vi "MB Serial Example Slave MK2.vi"() -> ()   [LabVIEW 2021]
uses:
  API/Wrapper/API Main.lvlib
  API/Slave/Modbus Slave.lvclass
  API/Wrapper/Create Serial Slave.vi
  Data Model/Identification Parameters.ctl
  Data Model/Device Data Model.lvclass
  Master Function Definition/Read Device ID code.ctl
panel:
  in  "VISA resource name":refnum<visa-resource-name>="COM8"
  in  "HR to write":u16[](array[numeric])=[1, 65535, 40000, 20000]
  in  "Set HR":bool
  in  "Set IR":bool
  in  "IR to write":u16[](array[numeric])=[1, 65535, 40000, 20000]
  in  "IR 6":u16
  in  "Set !":bool
  in  "! status":u8=1
  in  "Set Coils":bool
  in  "Set DI":bool
  in  "DI to write":bool[](array[boolean])=[FALSE, TRUE, FALSE, TRUE]
  in  "coils to write":bool[](array[boolean])=[FALSE, TRUE, FALSE, TRUE]
  in  "set objects":bool
  in  "Objects In":T1[](array[typedef])=[{"Object ID"=0, "Value"="National instruments"}, {"Object ID"=1, "Value"="42"}, {"Object ID"=2, "Value"="1.0.0"}] {"Object ID" format="%x"}
  in  "Coil 6":bool
  out "exception status":u8=1
  out "register values":u16[](array[numeric])=[1, 1, 65535, 40000, 20000, 6]
  out "discrete inputs":bool[](array[boolean])=[FALSE, FALSE, TRUE, FALSE, TRUE, TRUE]
  in  "Read Device ID code":T2
  out "Objects":T1[](array[typedef])=[{"Object ID"=0, "Value"="National instruments"}, {"Object ID"=1, "Value"="42"}, {"Object ID"=2, "Value"="1.0.0"}] {"Object ID" format="%x"}
  in  "Object Id":u8 format="%02x"
  out "holding reg":u16[](array[numeric])=[1, 1, 65535, 40000, 20000, 6]
  out "error out":errorcluster
  in  "stop":bool
  out "Coils":bool[](array[boolean])=[FALSE, FALSE, TRUE, FALSE, TRUE, TRUE] caption="Coils (Master can write coils)"
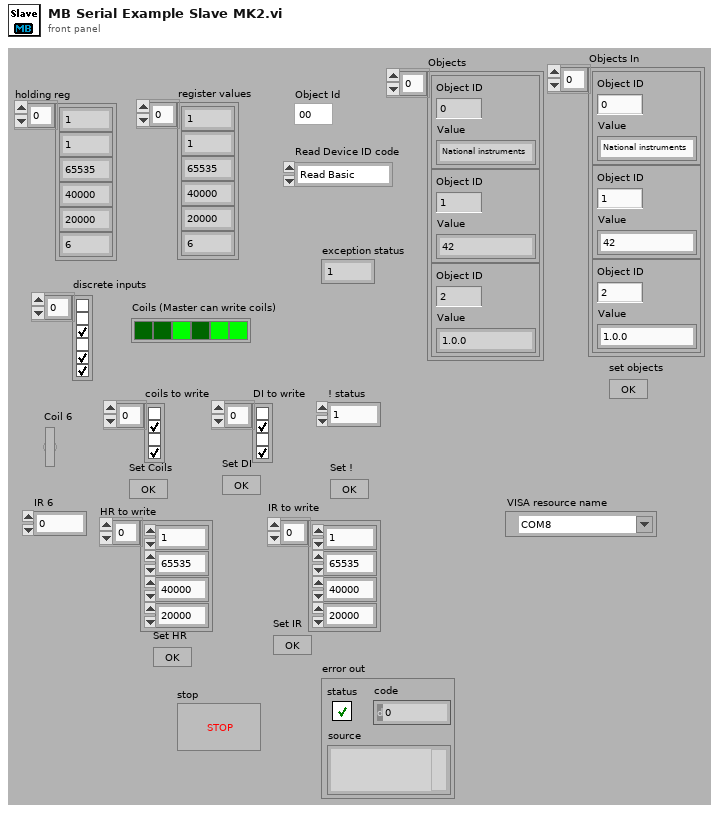
[diagram p1: front panel]
types:
  T1 = typedef "Device Data Model.lvclass/Identification Parameters.ctl" = cluster{"Object ID":u8, "Value":string}
  T2 = typedef "Device Data Model.lvclass/Read Device ID code.ctl" = enum8{"Read Basic", "Read Regular", "Read Extended", "Read Specific"}
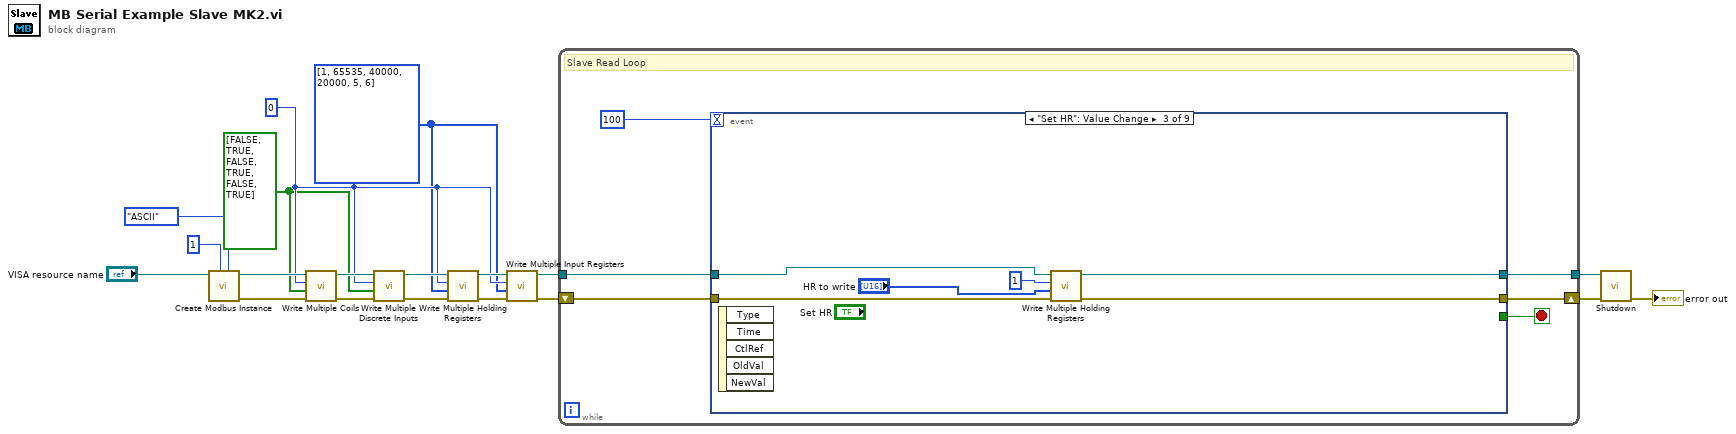
[diagram p0: block diagram]
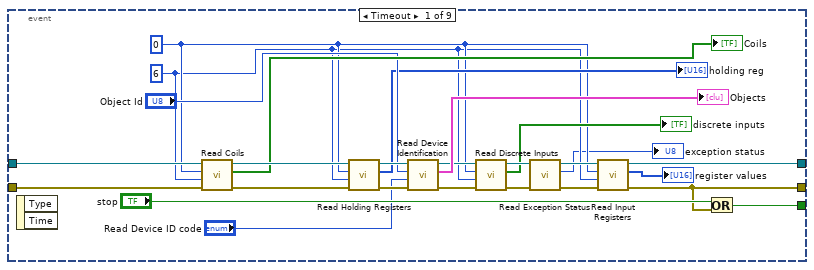
[diagram p2: hidden frame]
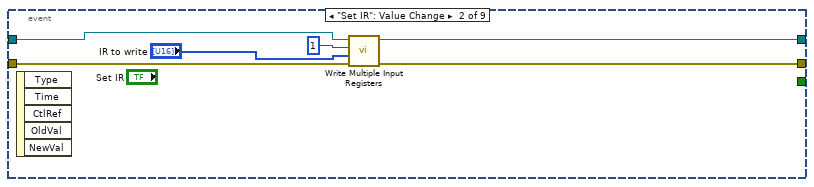
[diagram p3: hidden frame]
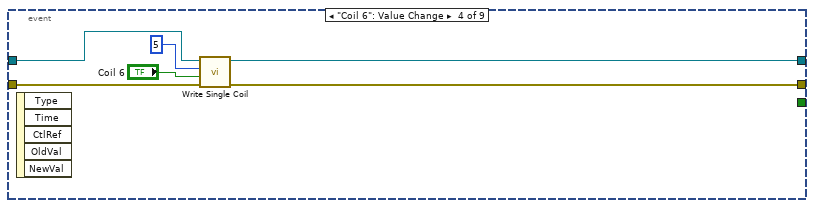
[diagram p4: hidden frame]
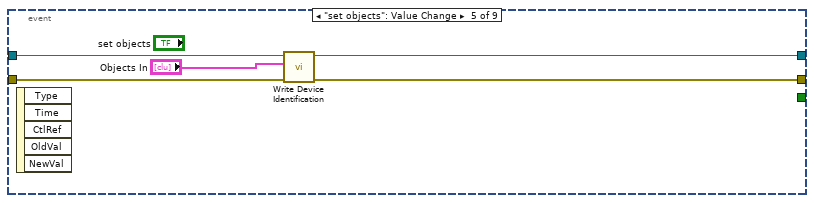
[diagram p5: hidden frame]
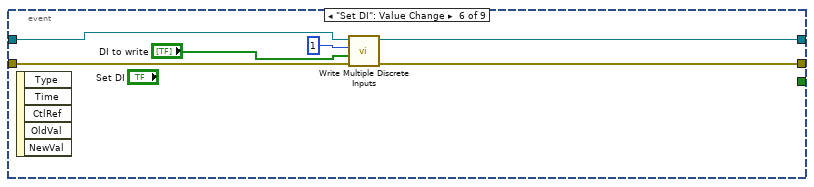
[diagram p6: hidden frame]
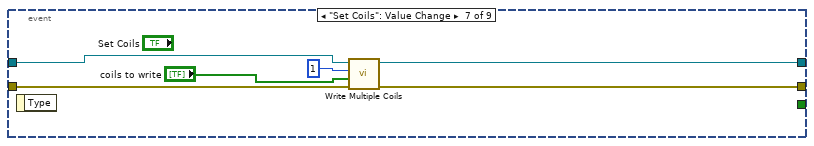
[diagram p7: hidden frame]
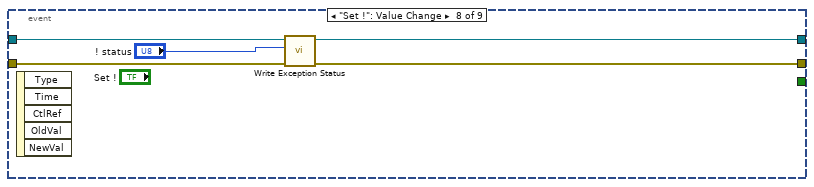
[diagram p8: hidden frame]
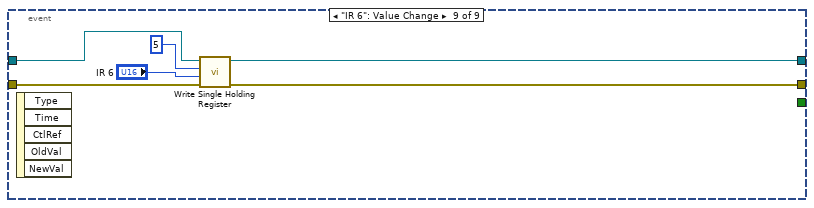
[diagram p9: hidden frame]
diagram:
  w4 = bool[] [FALSE, TRUE, FALSE, TRUE, FALSE, TRUE] ("coils to write")
  w5 = u16[] [1, 65535, 40000, 20000, 5, 6] ("registers")
  w6 = u16 0 ("starting address")
  n1 = call-poly "Create Modbus Instance.vi"("serial type"=enum16{"RTU", "ASCII"}."ASCII" ("Serial Type"), "unit ID"=u8 1 ("Unit ID"), "VISA resource name"="VISA resource name") -> ("error out"=w10:errorcluster, "serial slave instance"=w11:refnum<class "Modbus Slave.lvclass">)  [unwired: 7 in]
  n2 = call-dynamic "Write Multiple Coils.vi"("error in (no error)"=w10, "coil values"=w4, "starting address"=w6, "Modbus slave in"=w11) -> ("error out"=w9:errorcluster, "Modbus slave out"=w12:refnum<class "Modbus Slave.lvclass">)  [unwired: 6 in]
  n3 = call-dynamic "Write Multiple Discrete Inputs.vi"("error in (no error)"=w9, "discrete input values"=w4, "starting address"=w6, "Modbus slave in"=w12) -> ("error out"=w14:errorcluster, "Modbus slave out"=w13:refnum<class "Modbus Slave.lvclass">)  [unwired: 6 in]
  n4 = call-dynamic "Write Multiple Holding Registers.vi"("error in (no error)"=w14, "holding register values"=w5, "starting address"=w6, "Modbus slave in"=w13) -> ("error out"=w15:errorcluster, "Modbus slave out"=w16:refnum<class "Modbus Slave.lvclass">)  [unwired: 6 in]
  n5 = call-dynamic "Write Multiple Input Registers.vi"("error in (no error)"=w15, "input register values"=w5, "starting address"=w6, "Modbus slave in"=w16) -> ("error out"=w8:errorcluster, "Modbus slave out"=w7:refnum<class "Modbus Slave.lvclass">)  [unwired: 6 in]
  n6 = while {
    tunnel: [w21] -> w19
    tunnel: w7 -> [w24]
    shift-right: [w22] -> w18
    shift-left: w8 -> [w23]
    stop <- w25 stop-if-true
    # "Slave Read Loop"
    n7 = event shown="[2] \"Set HR\": Value Change" {
      selector: _ -> [_ _ _ _ _ _ _ _ _]
      dyn-events: _ -> [_ _ _ _ _ _ _ _ _]
      timeout: 100 -> [_ _ _ _ _ _ _ _ _]
      tunnel: [w48 _ _ _ _ _ _ _ _] -> w25
      tunnel: w24 -> [w43 w54 w63 w66 w71 w80 w83 w90 w97]
      tunnel: w23 -> [w42 w55 w60 w67 w72 w79 w84 w91 w96]
      tunnel: [w38 w56 w61 w68 w73 w76 w85 w88 w95] -> w22
      tunnel: [w37 w57 w62 w69 w74 w75 w86 w87 w94] -> w21
      event Timeout {
        w28 = u16 6 ("Number of coils")
        w29 = u16 0 ("Starting Address")
        n8 = event-data() -> ()  [unwired: 1 in, 2 out]
        n9 = call-dynamic "Read Coils.vi"("error in (no error)"=w42, "number of coils"=w28, "starting address"=w29, "Modbus slave in"=w43) -> ("error out"=w47:errorcluster, "coil values"=→"Coils":bool[], "Modbus slave out"=w46:refnum<class "Modbus Slave.lvclass">)  [unwired: 5 in]
        n10 = call-dynamic "Read Holding Registers.vi"("error in (no error)"=w47, "number of holding registers"=w28, "starting address"=w29, "Modbus slave in"=w46) -> ("error out"=w49:errorcluster, "register values"=→"holding reg":u16[], "Modbus slave out"=w50:refnum<class "Modbus Slave.lvclass">)  [unwired: 5 in]
        n11 = call-dynamic "Read Device Identification.vi"("error in (no error)"=w49, "read device ID code"="Read Device ID code", "object ID"="Object Id", "Modbus slave in"=w50) -> ("error out"=w34:errorcluster, "objects"=→"Objects":cluster{"object ID":u8, "value":string}[], "Modbus slave out"=w31:refnum<class "Modbus Slave.lvclass">)  [unwired: 5 in]
        n12 = call-dynamic "Read Discrete Inputs.vi"("error in (no error)"=w34, "number of discrete inputs"=w28, "starting address"=w29, "Modbus slave in"=w31) -> ("error out"=w35:errorcluster, "discrete input values"=→"discrete inputs":bool[], "Modbus slave out"=w33:refnum<class "Modbus Slave.lvclass">)  [unwired: 5 in]
        n13 = call-dynamic "Read Exception Status.vi"("error in (no error)"=w35, "Modbus slave in"=w33) -> ("error out"=w36:errorcluster, "exception status"=→"exception status":u8, "Modbus slave out"=w32:refnum<class "Modbus Slave.lvclass">)  [unwired: 7 in]
        n14 = call-dynamic "Read Input Registers.vi"("error in (no error)"=w36, "number of input registers"=w28, "starting address"=w29, "Modbus slave in"=w32) -> ("error out"=w38:errorcluster, "register values"=→"register values":u16[], "Modbus slave out"=w37:refnum<class "Modbus Slave.lvclass">)  [unwired: 5 in]
        n15 = Or(x="stop", y=w38) -> (x .or. y?=w48:bool)
      }
      event "Set IR": Value Change {
        n16 = event-data() -> ()  [unwired: 1 in, 5 out]
        n17 = call-dynamic "Write Multiple Input Registers.vi"("error in (no error)"=w55, "input register values"="IR to write", "starting address"=u16 1, "Modbus slave in"=w54) -> ("error out"=w56:errorcluster, "Modbus slave out"=w57:refnum<class "Modbus Slave.lvclass">)  [unwired: 6 in]
      }
      event "Set HR": Value Change {
        n18 = event-data() -> ()  [unwired: 1 in, 5 out]
        n19 = call-dynamic "Write Multiple Holding Registers.vi"("error in (no error)"=w60, "holding register values"="HR to write", "starting address"=u16 1, "Modbus slave in"=w63) -> ("error out"=w61:errorcluster, "Modbus slave out"=w62:refnum<class "Modbus Slave.lvclass">)  [unwired: 6 in]
      }
      event "Coil 6": Value Change {
        n20 = event-data() -> ()  [unwired: 1 in, 5 out]
        n21 = call-dynamic "Write Single Coil.vi"("error in (no error)"=w67, "coil value"="Coil 6", "address"=u16 5, "Modbus slave in"=w66) -> ("error out"=w68:errorcluster, "Modbus slave out"=w69:refnum<class "Modbus Slave.lvclass">)  [unwired: 6 in]
      }
      event "set objects": Value Change {
        n22 = event-data() -> ()  [unwired: 1 in, 5 out]
        n23 = call-dynamic "Write Device Identification.vi"("error in (no error)"=w72, "objects"="Objects In", "Modbus slave in"=w71) -> ("error out"=w73:errorcluster, "Modbus slave out"=w74:refnum<class "Modbus Slave.lvclass">)  [unwired: 7 in]
      }
      event "Set DI": Value Change {
        n24 = event-data() -> ()  [unwired: 1 in, 5 out]
        n25 = call-dynamic "Write Multiple Discrete Inputs.vi"("error in (no error)"=w79, "discrete input values"="DI to write", "starting address"=u16 1, "Modbus slave in"=w80) -> ("error out"=w76:errorcluster, "Modbus slave out"=w75:refnum<class "Modbus Slave.lvclass">)  [unwired: 6 in]
      }
      event "Set Coils": Value Change {
        n26 = event-data() -> ()  [unwired: 1 in, 1 out]
        n27 = call-dynamic "Write Multiple Coils.vi"("error in (no error)"=w84, "coil values"="coils to write", "starting address"=u16 1, "Modbus slave in"=w83) -> ("error out"=w85:errorcluster, "Modbus slave out"=w86:refnum<class "Modbus Slave.lvclass">)  [unwired: 6 in]
      }
      event "Set !": Value Change {
        n28 = event-data() -> ()  [unwired: 1 in, 5 out]
        n29 = call "Write Exception Status.vi"("error in (no error)"=w91, "exception status"="! status", "Modbus slave in"=w90) -> ("error out"=w88:errorcluster, "Modbus slave out"=w87:refnum<class "Modbus Slave.lvclass">)  [unwired: 7 in]
      }
      event "IR 6": Value Change {
        n30 = event-data() -> ()  [unwired: 1 in, 5 out]
        n31 = call-dynamic "Write Single Holding Register.vi"("error in (no error)"=w96, "holding register value"="IR 6", "address"=u16 5, "Modbus slave in"=w97) -> ("error out"=w95:errorcluster, "Modbus slave out"=w94:refnum<class "Modbus Slave.lvclass">)  [unwired: 6 in]
      }
    }
  }
  n32 = call-dynamic "Shutdown.vi"("error in (no error)"=w18, "Modbus slave in"=w19) -> ("error out"=→"error out":errorcluster)  [unwired: 9 in]
